vi "Class to Variant.vi"(8 "error in (no error)":errorcluster, 10 "Data in":variant, 11 "Job Initialize in":refnum<class "Job Initialize.lvclass">) -> (0 "error out":errorcluster, 1 "Serialized Object Name":string, 2 "Data Out":variant, 3 "Job Initialize out":refnum<class "Job Initialize.lvclass">)   [LabVIEW 2014, in "Job Initialize.lvclass"]
uses:
  Job Initialize.lvclass
  Job Initialize.lvclass/Job Initialize.ctl
  Build Job/Build Job.lvclass
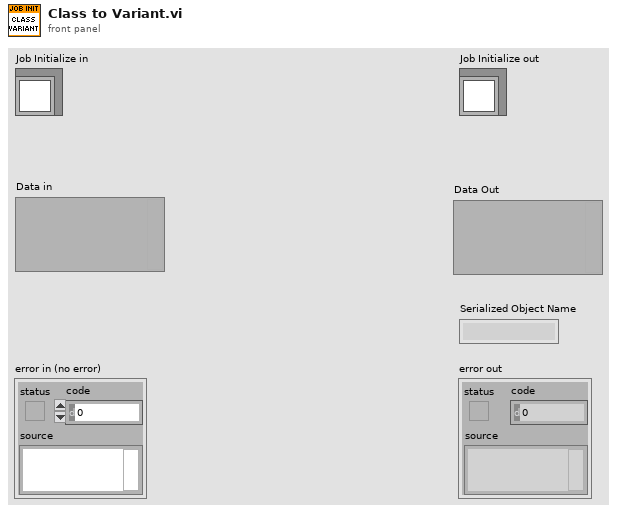
[diagram p1: front panel]
types:
  T1 = typedef "Source Code Control Selection - STYP.ctl" = enum16{"None (Manual Build)", "Every 15 Minutes", "Every 30 Minutes", "Every 45 Minutes", "Every Hour", "Every 2 Hours", "Everyday "}
  T2 = typedef "Cron String - STYP.ctl" = cluster{"Day of Week":enum16{"Everyday", "Sunday", "Monday", "Tuesday", "Wednesday", "Thursday", "Friday", "Saturday"}, "Hour":i32, "Enable?":bool}
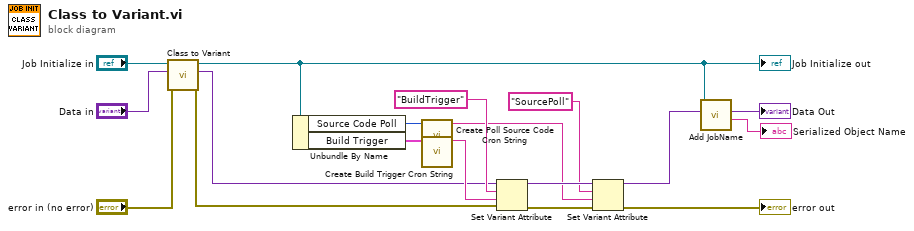
[diagram p0: block diagram]
diagram:
  n1 = call-parent "Class to Variant.vi"("error in (no error)"="error in (no error)", "Data in"="Data in", "Build Job in"="Job Initialize in") -> ("error out"=w7:errorcluster, "Data Out"=w8:variant, "Build Job out"=w4:refnum<class "Job Initialize.lvclass">)  [unwired: 5 in, 1 out]
  "Job Initialize out" <- w4
  n2 = Unbundle By Name(w4) -> ("Source Code Poll"=w10:T1, "Build Trigger"=w12:T2)
  n3 = call "Create Poll Source Code Cron String.vi"("Source Code Poll"=w10) -> ("String"=w9:string)  [unwired: 10 in]
  n4 = call "Create Build Trigger Cron String.vi"("Cron"=w12) -> ("String"=w11:string)  [unwired: 10 in]
  n5 = Set Variant Attribute(Variant=w8, name="BuildTrigger", value=w11, error in=w7) -> (Variant out=w15:variant, error out=w14:errorcluster)  [unwired: 1 out]
  n6 = Set Variant Attribute(Variant=w15, name="SourcePoll", value=w9, error in=w14) -> (Variant out=w5:variant, error out=→"error out":errorcluster)  [unwired: 1 out]
  n7 = call "Add JobName.vi"("Data in"=w5, "Build Job in"=w4) -> ("Job Name"=→"Serialized Object Name":string, "Data Out"=→"Data Out":variant)  [unwired: 8 in]
